vi "TharClose.vi"(8 "error in (no error)":errorcluster, 11 "Handle":u32) -> (0 "error out":errorcluster)   [LabVIEW 2016]
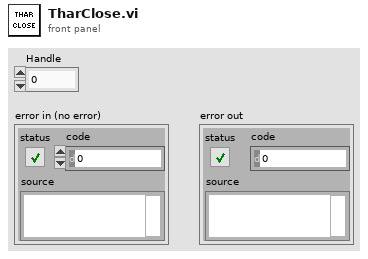
[diagram p1: front panel]
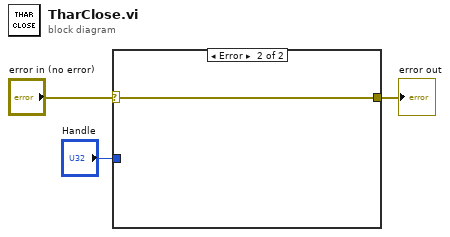
[diagram p0: block diagram]
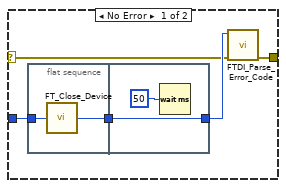
[diagram p2: hidden frame]
diagram:
  n1 = case shown="Error" "error in (no error)" {
    selector: "error in (no error)" -> [w4 w13]
    tunnel: [w8 w13] -> w3
    tunnel: "Handle" -> [w6 _]
    frame No Error {
      n2 = flat-sequence {
        tunnel: w6 -> [w9]
        tunnel: [w10] -> w5
        tunnel: [w12] -> w7
        tunnel: w5 -> [w12]
        frame #0 {
          n3 = call "FT_Close_Device.vi"("Handle"=w9) -> ("FT_Status"=w10:u32)
        }
        frame #1 {
          n4 = Wait (ms)(milliseconds to wait=u32 50) -> ()  [unwired: 1 out]
        }
      }
      n5 = call "FTDI_Parse_Error_Code.vi"("error in (no error)"=w4, "FT_Status"=w7) -> ("error out"=w8:errorcluster)  [unwired: 9 in]
    }
    frame Error {
    }
  }
  "error out" <- w3
